vi "Main.vi"() -> ()   [LabVIEW 2014]
uses:
  <vilib>/ethernetip/ethernetip.llb/EthernetIP Tag Write BOOL.vi
  <vilib>/ethernetip/ethernetip.llb/EthernetIP Tag Write REAL.vi
  <vilib>/ethernetip/ethernetip.lvlib
  <vilib>/vision/driver/NI_Vision_Acquisition_Software.lvlib
panel:
  in  "스피드":u32[](array[knob])=[80] scale=0.0..100.0
  in  "부하 제한 값":u32(slide)=70 scale=0.0..100.0
  out "위치 그래프":dbl[][](graph)
  in  "시간 지연":u32(slide)=200 scale=0.0..900.0
  in  "Error In":errorcluster
  in  "우측 위치 값":u32[](array[knob])=[35] scale=0.0..100.0
  in  "좌측 위치 값":u32[](array[knob])=[40] scale=0.0..100.0
  out "Axis":string="L127R127C127"
  in  "포트":u16=50
  in  "IP":string="127.0.0.1"
  in  "Running Game":string="DiRT 3"
  out "Loop Count":i32=6322
  in  "Error RESET":bool
  in  "Simtools ON":bool=TRUE
  in  "Motor Start":bool
  in  "Motor Reset":bool
  in  "STOP":bool
  in  "DOF OFF":bool
  in  "DOF ON":bool
  out "Running":bool
  out "Error Out":errorcluster
  # "지도교수 : 손종원 교수님, 노일수 교수님    개발자 : 하기봉, 박재우"
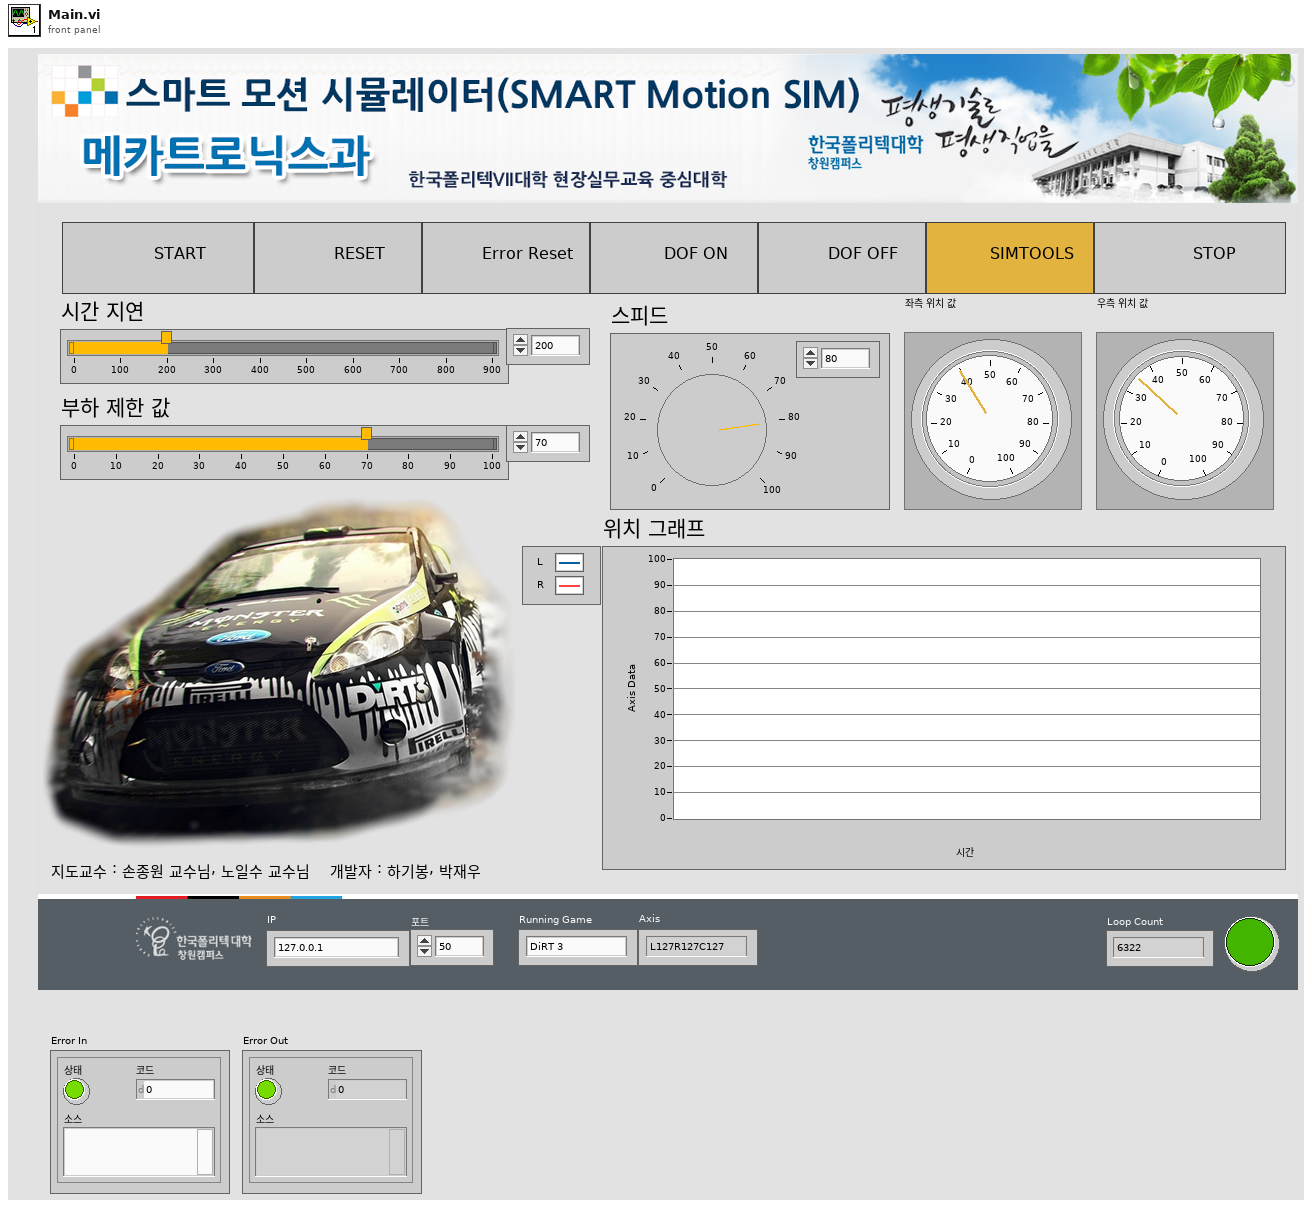
[diagram p1: front panel]
types:
  T1 = typedef "IMAQdx.ctl" = refnum<k21>
  T2 = typedef "IMAQ Image.ctl" = refnum<image>
  T3 = typedef "ethernetip.lvlib/ethernetip.ctl" = refnum<k21>
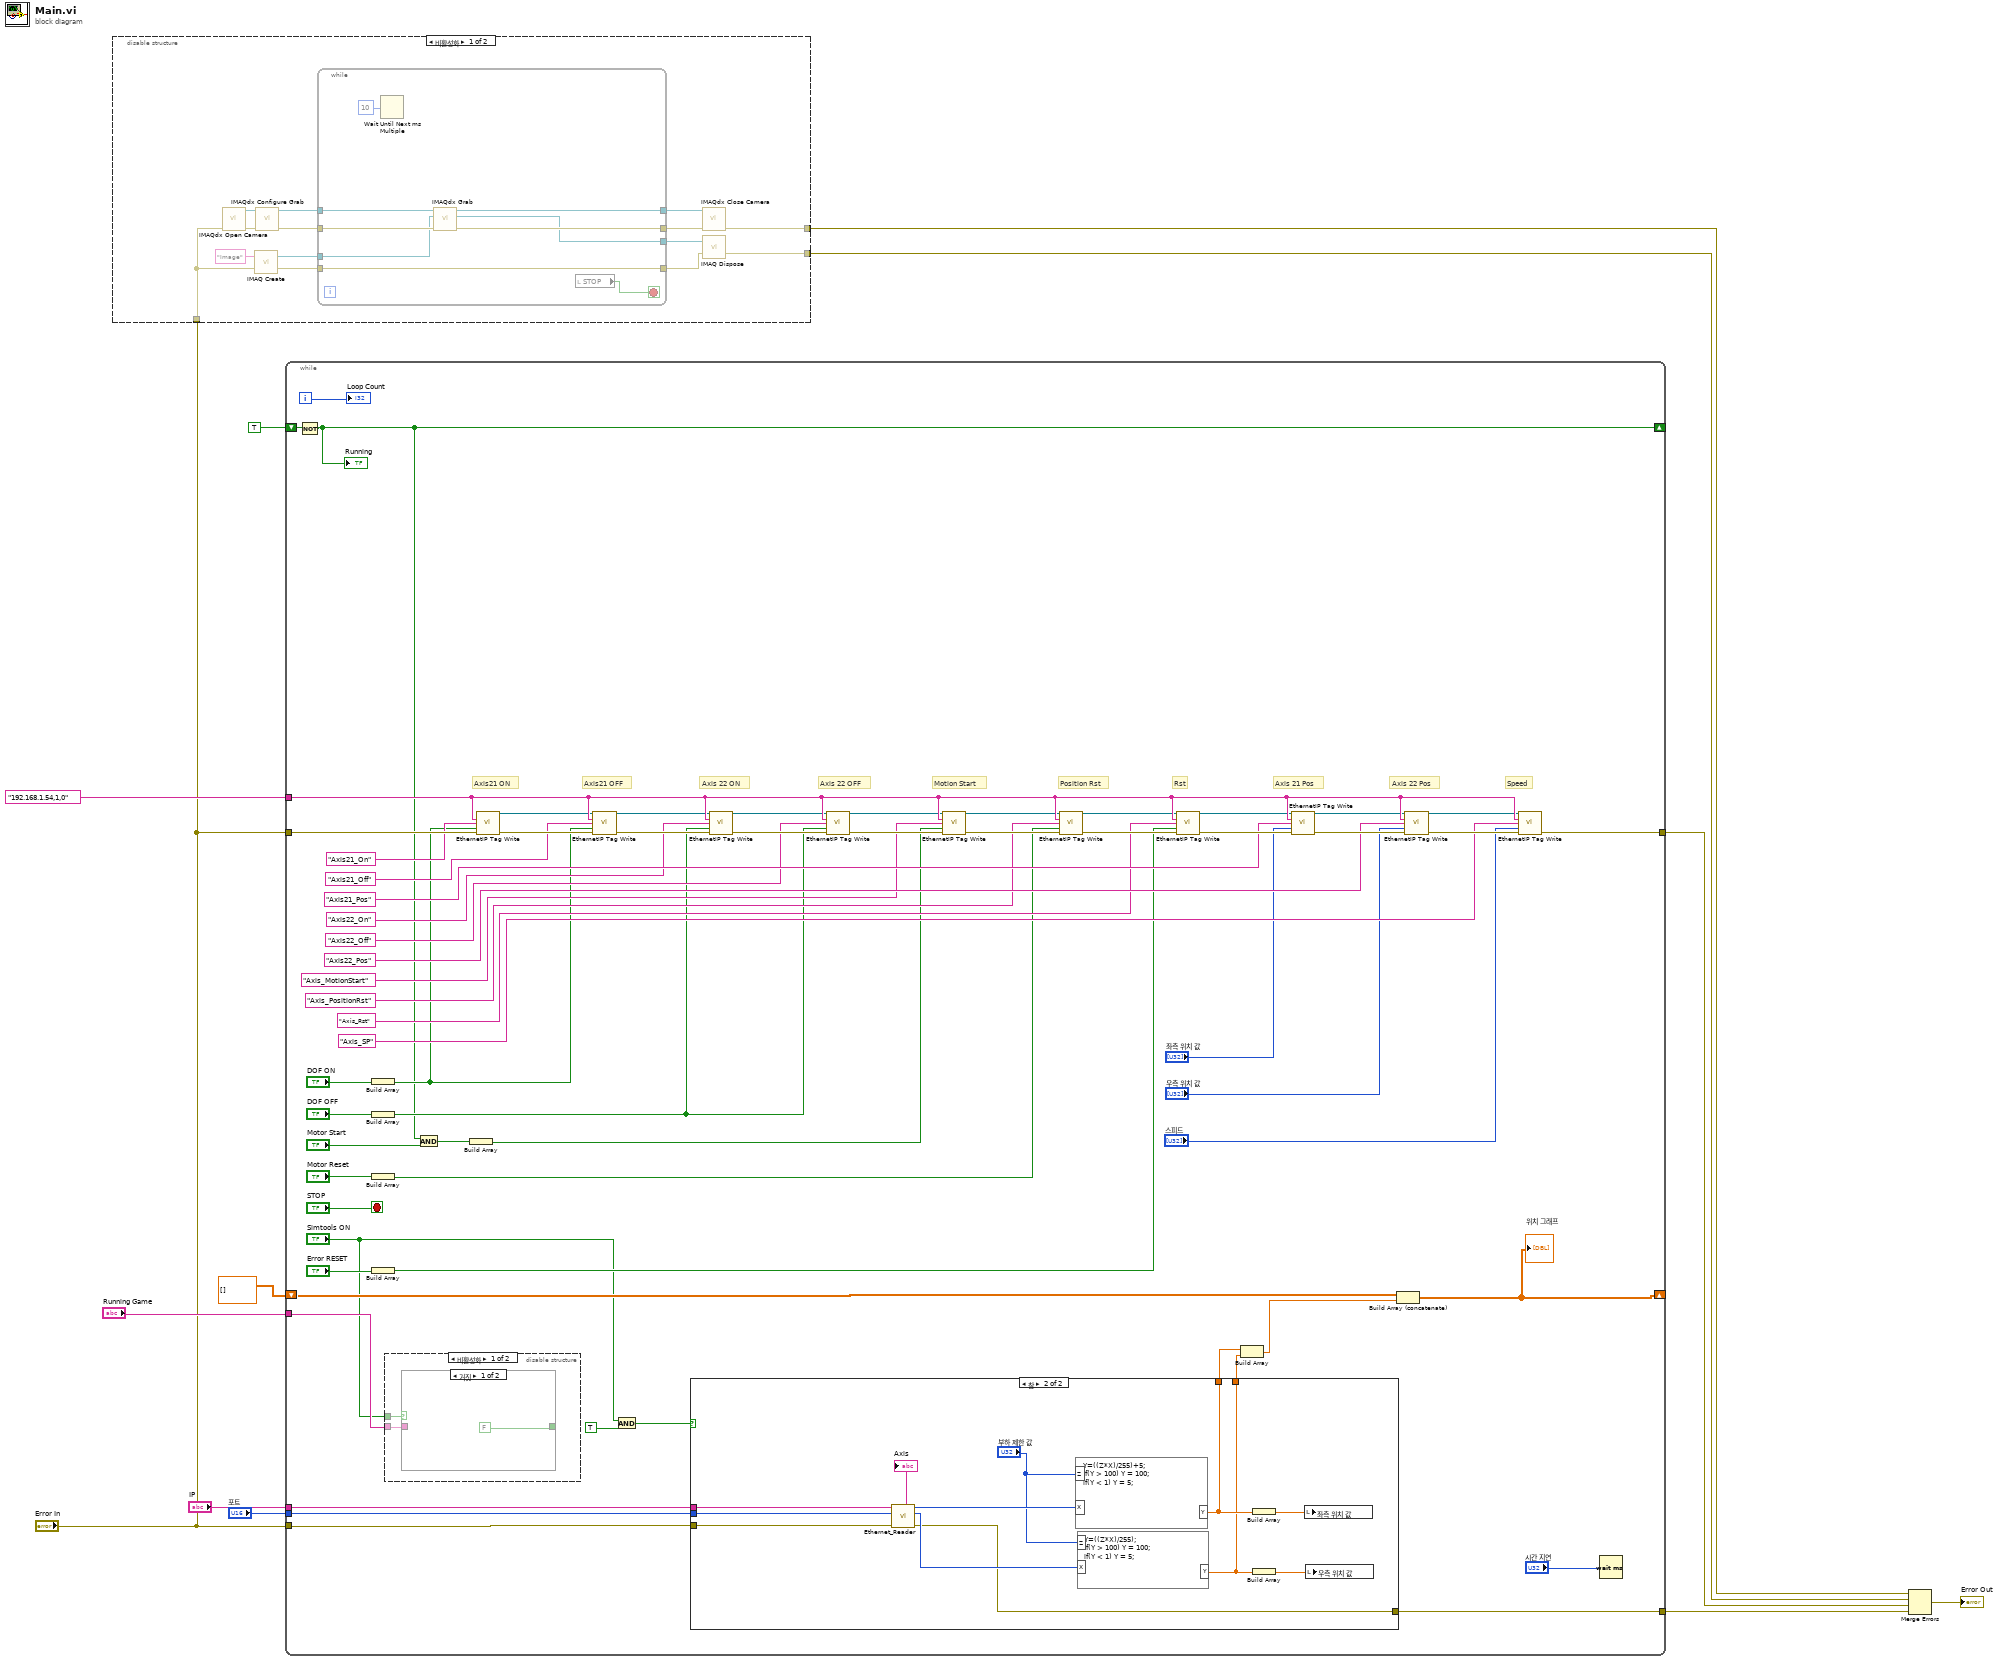
[diagram p0: block diagram]
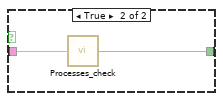
[diagram p3: hidden frame]
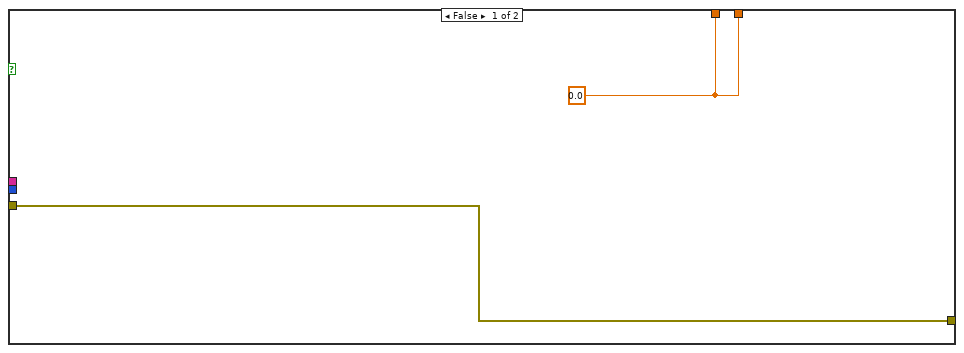
[diagram p5: hidden frame]
diagram:
  n1 = disable-structure shown="비활성화" {
    disable-tunnel: [w23 _] -> w6
    disable-tunnel: [w22 _] -> w5
    disable-tunnel: "Error In" -> [w21 _]
    frame Disabled {
      n2 = call <vilib>:"IMAQdx Open Camera.vi"("error in"=w21) -> ("error out"=w25:errorcluster, "Session Out"=w26:T1, "Session In"=w27:T1)  [unwired: 8 in]
      n3 = call "IMAQ Create"("Image Name"="Image", "error in (no error)"=w21) -> ("New Image"=w16:T2, "error out"=w14:errorcluster)  [unwired: 3 in]
      n4 = call <vilib>:"IMAQdx Configure Grab.vi"("error in"=w25, "Session In"=w26) -> ("error out"=w20:errorcluster, "Session Out"=w18:T1)  [unwired: 8 in]
      n5 = while {
        tunnel: w20 -> [w36]
        tunnel: [w35] -> w19
        tunnel: w18 -> [w34]
        tunnel: [w33] -> w17
        tunnel: w16 -> [w32]
        tunnel: [w31] -> w15
        tunnel: w14 -> [w31]
        tunnel: [w30] -> w13
        stop <- w29 stop-if-true
        n6 = Wait Until Next ms Multiple(millisecond multiple=u32 10 ("ms 배수")) -> ()  [unwired: 1 out]
        n7 = call <vilib>:"IMAQdx Grab.vi"("error in"=w36, "Image In"=w32, "Session In"=w34) -> ("error out"=w35:errorcluster, "Image Out"=w30:T2, "Session Out"=w33:T1)  [unwired: 5 in, 1 out]
        n8 = local read "STOP"() -> (w29:bool)
      }
      n9 = call <vilib>:"IMAQdx Close Camera.vi"("error in"=w19, "Session In"=w17) -> ("error out"=w22:errorcluster)  [unwired: 9 in]
      n10 = call "IMAQ Dispose"("Image"=w13, "error in (no error)"=w15) -> ("error out"=w23:errorcluster)  [unwired: 4 in]
    }
    frame Enabled {
    }
  }
  n11 = while {
    tunnel: "Error In" -> [w99]
    tunnel: [w89] -> w7
    tunnel: "192.168.1.54,1,0" ("Network Path") -> [w88]
    shift-right: [w40] -> _
    shift-left: TRUE -> [w41]
    tunnel: "Running Game" -> [w50]
    tunnel: "포트" -> [w54]
    tunnel: "IP" -> [w53]
    tunnel: "Error In" -> [w52]
    tunnel: [w51] -> w2
    shift-right: [w45] -> _
    shift-left: dbl[][] [] -> [w48]
    i -> [w56]
    stop <- "STOP" stop-if-true
    # "Speed"
    # "Rst"
    # "Position Rst"
    # "Motion Start"
    # "Axis 22 Pos"
    # "Axis 22 OFF"
    # "Axis 22 ON"
    # "Axis 21 Pos"
    # "Axis21 OFF"
    # "Axis21 ON"
    n12 = Not(x=w41) -> (.not. x?=w40:bool)
    "Running" <- w40
    n13 = Build Array("DOF ON") -> (w62:bool[])
    n14 = Build Array("DOF OFF") -> (w61:bool[])
    n15 = Build Array("Motor Reset") -> (w59:bool[])
    n16 = Build Array("Error RESET") -> (w57:bool[])
    n17 = disable-structure shown="비활성화" {
      disable-tunnel: w50 -> [w101 _]
      disable-tunnel: "Simtools ON" -> [w100 _]
      frame Disabled {
        n18 = case shown="거짓" w100 {
          tunnel: w101 -> [_ w104]
          tunnel: [FALSE w103] -> _
          frame False {
          }
          frame True {
            n19 = call "Processes_check.vi"("검색 내용"=w104) -> ("불리언"=w103:bool)
          }
        }
      }
      frame Enabled {
      }
    }
    n20 = And(x=w40, y="Motor Start") -> (x .and. y?=w64:bool)
    n21 = Build Array(w64) -> (w63:bool[])
    n22 = call-poly <vilib>:"EthernetIP Tag Write.vi"("Network Path"=w88, "Tag Name"="Axis21_On", "Data"=w62, "error in"=w99) -> ("Session out"=w87:T3, "error out"=w98:errorcluster)  [unwired: 10 in]
    n23 = call-poly <vilib>:"EthernetIP Tag Write.vi"("Session in"=w87, "Network Path"=w88, "Tag Name"="Axis21_Off", "Data"=w62, "error in"=w98) -> ("Session out"=w86:T3, "error out"=w97:errorcluster)  [unwired: 9 in]
    n24 = And(x="Simtools ON", y=TRUE) -> (x .and. y?=w55:bool)
    n25 = case shown="참" w55 {
      tunnel: w54 -> [_ w115]
      tunnel: w53 -> [_ w114]
      tunnel: w52 -> [w106 w111]
      tunnel: [w106 w110] -> w51
      tunnel: [w105 w109] -> w43
      tunnel: [w105 w108] -> w42
      frame False {
        w105 = 0.0
      }
      frame True {
        n26 = call "Ethernet_Reader.vi"("에러 입력(에러 없음)"=w111, "포트"=w115, "IP"=w114) -> ("에러 출력"=w110:errorcluster, "R"=w116:u32, "L"=w117:u32, "Axis"=→"Axis":string)  [unwired: 5 in]
        n27 = formula code="Y=((Z*X)/255)+5;\nif(Y > 100) Y = 100;\nif(Y < 1) Y = 5;"("X"=w117, "Z"="부하 제한 값") -> ("Y"=w109:dbl)
        n28 = formula code="Y=((Z*X)/255);\nif(Y > 100) Y = 100;\nif(Y < 1) Y = 5;"("X"=w116, "Z"="부하 제한 값") -> ("Y"=w108:dbl)
        n29 = Build Array(w109) -> (w113:dbl[])
        n30 = Build Array(w108) -> (w112:dbl[])
        n31 = local write "좌측 위치 값"(w113) -> ()
        n32 = local write "우측 위치 값"(w112) -> ()
      }
    }
    n33 = call-poly <vilib>:"EthernetIP Tag Write.vi"("Session in"=w86, "Network Path"=w88, "Tag Name"="Axis22_On", "Data"=w61, "error in"=w97) -> ("Session out"=w85:T3, "error out"=w96:errorcluster)  [unwired: 9 in]
    n34 = call-poly <vilib>:"EthernetIP Tag Write.vi"("Session in"=w85, "Network Path"=w88, "Tag Name"="Axis22_Off", "Data"=w61, "error in"=w96) -> ("Session out"=w84:T3, "error out"=w95:errorcluster)  [unwired: 9 in]
    n35 = call-poly <vilib>:"EthernetIP Tag Write.vi"("Session in"=w84, "Network Path"=w88, "Tag Name"="Axis_MotionStart", "Data"=w63, "error in"=w95) -> ("Session out"=w83:T3, "error out"=w94:errorcluster)  [unwired: 9 in]
    n36 = call-poly <vilib>:"EthernetIP Tag Write.vi"("Session in"=w83, "Network Path"=w88, "Tag Name"="Axis_PositionRst", "Data"=w59, "error in"=w94) -> ("Session out"=w82:T3, "error out"=w93:errorcluster)  [unwired: 9 in]
    n37 = call-poly <vilib>:"EthernetIP Tag Write.vi"("Session in"=w82, "Network Path"=w88, "Tag Name"="Axis_Rst", "Data"=w57, "error in"=w93) -> ("Session out"=w81:T3, "error out"=w92:errorcluster)  [unwired: 9 in]
    n38 = Build Array(w43, w42) -> (w44:dbl[])
    n39 = call-poly <vilib>:"EthernetIP Tag Write.vi"("Session in"=w81, "Network Path"=w88, "Tag Name"="Axis21_Pos", "Data"="좌측 위치 값", "error in"=w92) -> ("Session out"=w80:T3, "error out"=w91:errorcluster)  [unwired: 9 in]
    n40 = Build Array (concatenate)(w48, w44) -> (w45:dbl[][])
    "위치 그래프" <- w45
    n41 = call-poly <vilib>:"EthernetIP Tag Write.vi"("Session in"=w80, "Network Path"=w88, "Tag Name"="Axis22_Pos", "Data"="우측 위치 값", "error in"=w91) -> ("Session out"=w79:T3, "error out"=w90:errorcluster)  [unwired: 9 in]
    n42 = call-poly <vilib>:"EthernetIP Tag Write.vi"("Session in"=w79, "Network Path"=w88, "Tag Name"="Axis_SP", "Data"="스피드", "error in"=w90) -> ("error out"=w89:errorcluster)  [unwired: 9 in, 1 out]
    n43 = Wait (ms)(milliseconds to wait="시간 지연") -> ()  [unwired: 1 out]
    "Loop Count" <- w56
  }
  n44 = Merge Errors(w5, w6, w7, w2) -> (→"Error Out":errorcluster)
